vi "MGCC_MdlMgmt_MovetonewMicrogrid.vi"() -> ()   [LabVIEW 2016]
doc: "-----------------------------------------------------------------------------------------------------------------------\nCopyright <2019> <The University of Tennessee at Knoxville and the University of Tennessee Research Foundation>\nThis software is released under BSD-3 \nhttps://opensource.org/licenses/BSD-3-Clause \nAdditional license options available at https://utrf.tennessee.edu/industry/sample-agreements/\n-----------------------------------------------------------------------------------------------------------------------"
uses:
  Global_MdlMgmt.vi
  <vilib>/imath/engines/lvmath2/RunTimeEngine/IndexRead/NIMS M($,R2).vi
  <instcachedir>/0/NIMS M($,R2)_D9380E19261A4ADFB2D364AF6959C6EF.lvgen/NIMS M($,R2)_D9380E19261A4ADFB2D364AF6959C6EF_001.vi
  <vilib>/imath/engines/lvmath2/RunTimeEngine/BuiltInFunctions/max/1 input/NIMS_max(RM).vi
  <instcachedir>/0/NIMS_max(RM)_358AE92FF7FA4D91BF0D9DEC69043403.lvgen/NIMS_max(RM)_358AE92FF7FA4D91BF0D9DEC69043403_000.vi
  <vilib>/imath/engines/lvmath2/RunTimeEngine/BuiltInFunctions/max/1 input/NIMS_max(RV).vi
  <instcachedir>/0/NIMS_max(RV)_237633DB1D604D5BA7001287DF3C7957.lvgen/NIMS_max(RV)_237633DB1D604D5BA7001287DF3C7957_000.vi
  <vilib>/imathl/engines/lvmath/Functions/Error Handling/Create Error.vi
  <vilib>/imath/engines/lvmath2/RunTimeEngine/IndexRead/NIMS M($,S).vi
  <instcachedir>/0/NIMS M($,S)_3E5749BBB62E49528D4765A77F1F6D98.lvgen/NIMS M($,S)_3E5749BBB62E49528D4765A77F1F6D98_000.vi
  <vilib>/imath/engines/lvmath2/RunTimeEngine/BuiltInFunctions/length/NIMS_length(GV).vi
  <instcachedir>/0/NIMS_length(GV)_08A3D13377FD4E4B96F5795FBF3698FA.lvgen/NIMS_length(GV)_08A3D13377FD4E4B96F5795FBF3698FA_000.vi
  <instcachedir>/0/NIMS_length(GV)_08A3D13377FD4E4B96F5795FBF3698FA.lvgen/NIMS_length(GV)_08A3D13377FD4E4B96F5795FBF3698FA_002.vi
  <vilib>/imath/engines/lvmath2/RunTimeEngine/BuiltInFunctions/zeros/NIMS_M=zeros(I32,I32).vi
  <vilib>/imath/engines/lvmath2/RunTimeEngine/ErrorHandling/NIMS_Create Error From Enums.vi
  <vilib>/imath/engines/lvmath2/RunTimeEngine/IndexReplace/NIMS M(S,$)=V.vi
  <instcachedir>/0/NIMS M(S,$)=V_BCCFA522A894489B8FA760383D74A164.lvgen/NIMS M(S,$)=V_BCCFA522A894489B8FA760383D74A164_002.vi
  <vilib>/imath/engines/lvmath2/RunTimeEngine/BuiltInFunctions/zeros/NIMS_V=zeros(I32,I32).vi
  <vilib>/imath/engines/lvmath2/RunTimeEngine/RangeToken/NIMS_Range_R3 - Integer.vi
  <instcachedir>/0/NIMS_Range_R3 - Integer_A435E2FF893B4C718FD5055FE39FE2F6.lvgen/NIMS_Range_R3 - Integer_A435E2FF893B4C718FD5055FE39FE2F6_000.vi
  <vilib>/imath/engines/lvmath2/RunTimeEngine/CommandStatement/MC_CommandStatement_break.vi
  <vilib>/imath/engines/lvmath2/RunTimeEngine/IndexRead/NIMS M(S,R2).vi
  <instcachedir>/0/NIMS M(S,R2)_45730E4D0DB74D118F715F4F99DCE4D7.lvgen/NIMS M(S,R2)_45730E4D0DB74D118F715F4F99DCE4D7_000.vi
  <vilib>/imath/engines/lvmath2/RunTimeEngine/BuiltInFunctions/is_membermx/NIMS_is_membermx(GM,GM).vi
  <instcachedir>/0/NIMS_is_membermx(GM,GM)_DE25F6F493CE4EA1946032CBAF7A49B3.lvgen/NIMS_is_membermx(GM,GM)_DE25F6F493CE4EA1946032CBAF7A49B3_000.vi
  <vilib>/imath/engines/lvmath2/RunTimeEngine/BuiltInFunctions/sum/NIMS_sum(GM,Sca).vi
  <instcachedir>/0/NIMS_sum(GM,Sca)_79BF37D5D11844228B167097B6AFCFEB.lvgen/NIMS_sum(GM,Sca)_79BF37D5D11844228B167097B6AFCFEB_001.vi
  <vilib>/imath/engines/lvmath2/RunTimeEngine/IndexRead/NIMS M(S,S).vi
  <instcachedir>/0/NIMS M(S,S)_AC51E74150A542F7991B9634C66F3096.lvgen/NIMS M(S,S)_AC51E74150A542F7991B9634C66F3096_000.vi
  <vilib>/imath/engines/lvmath2/RunTimeEngine/IndexReplace/NIMS M(S,S)=S.vi
  <instcachedir>/0/NIMS M(S,S)=S_98E40400474E4398B113AE20298B4F82.lvgen/NIMS M(S,S)=S_98E40400474E4398B113AE20298B4F82_000.vi
  <vilib>/imath/engines/lvmath2/RunTimeEngine/BuiltInFunctions/sum/NIMS_sum(GV).vi
  <instcachedir>/0/NIMS_sum(GV)_67F5EC36BC034E54A6BEC5B0673C00E5.lvgen/NIMS_sum(GV)_67F5EC36BC034E54A6BEC5B0673C00E5_000.vi
  <vilib>/imath/engines/lvmath2/RunTimeEngine/BuiltInFunctions/findnz/NIMS_[1o]_findnz(GRowV).vi
  <instcachedir>/0/NIMS_[1o]_findnz(GRowV)_1AF74843B4874134ADE908C0A4A72F3C.lvgen/NIMS_[1o]_findnz(GRowV)_1AF74843B4874134ADE908C0A4A72F3C_000.vi
  <vilib>/imath/engines/lvmath2/RunTimeEngine/IndexRead/NIMS M($,V).vi
  <instcachedir>/0/NIMS M($,V)_706F2CE2C8E141269FD4C8A402E169C5.lvgen/NIMS M($,V)_706F2CE2C8E141269FD4C8A402E169C5_005.vi
  <vilib>/imath/engines/lvmath2/RunTimeSupport/NIMS_Get Any Vector_w Error - Matrix.vi
  <instcachedir>/0/NIMS_Get Any Vector_w Error - Matrix_2B7BCBEFD1FA4E1C95EFF9244314B21B.lvgen/NIMS_Get Any Vector_w Error - Matrix_2B7BCBEFD1FA4E1C95EFF9244314B21B_001.vi
  <vilib>/imath/engines/lvmath2/RunTimeEngine/BuiltInFunctions/sets_union/NIMS_sets_union(GV2).vi
  <instcachedir>/0/NIMS_sets_union(GV2)_D04DE11E528744D2B40881BC08732835.lvgen/NIMS_sets_union(GV2)_D04DE11E528744D2B40881BC08732835_007.vi
  <vilib>/imath/engines/lvmath2/RunTimeEngine/IndexReplace/NIMS M($,V)=V.vi
  <instcachedir>/0/NIMS M($,V)=V_456DED019FC24BEA8A1C4EECB3220DB5.lvgen/NIMS M($,V)=V_456DED019FC24BEA8A1C4EECB3220DB5_000.vi
  <vilib>/imath/engines/lvmath2/RunTimeEngine/RangeToken/NIMS_Range.vi
  <instcachedir>/0/NIMS_Range_A7C094595B484CA7AF10685B02D808ED.lvgen/NIMS_Range_A7C094595B484CA7AF10685B02D808ED_001.vi
  <vilib>/imath/engines/lvmath2/RunTimeEngine/NodeEndStatement/NIMS_NodeEndStatement_Output.vi
  <instcachedir>/0/NIMS_NodeEndStatement_Output_53EC0D466D134D7ABD903AC30B43404B.lvgen/NIMS_NodeEndStatement_Output_53EC0D466D134D7ABD903AC30B43404B_002.vi
  <instcachedir>/0/NIMS_NodeEndStatement_Output_53EC0D466D134D7ABD903AC30B43404B.lvgen/NIMS_NodeEndStatement_Output_53EC0D466D134D7ABD903AC30B43404B_011.vi
  <vilib>/imath/engines/lvmath2/RunTimeEngine/ErrorHandling/NIMS_Finalize Error.vi
  <vilib>/Utility/error.llb/Error Cluster From Error Code.vi
  <vilib>/ErrorRing/Error Ring.xnode
panel:
  out "Nodematrix":dbl[][](array[numeric])
  out "island_number":i32
  out "Microgrid Topology Overall":dbl[][](array[numeric])
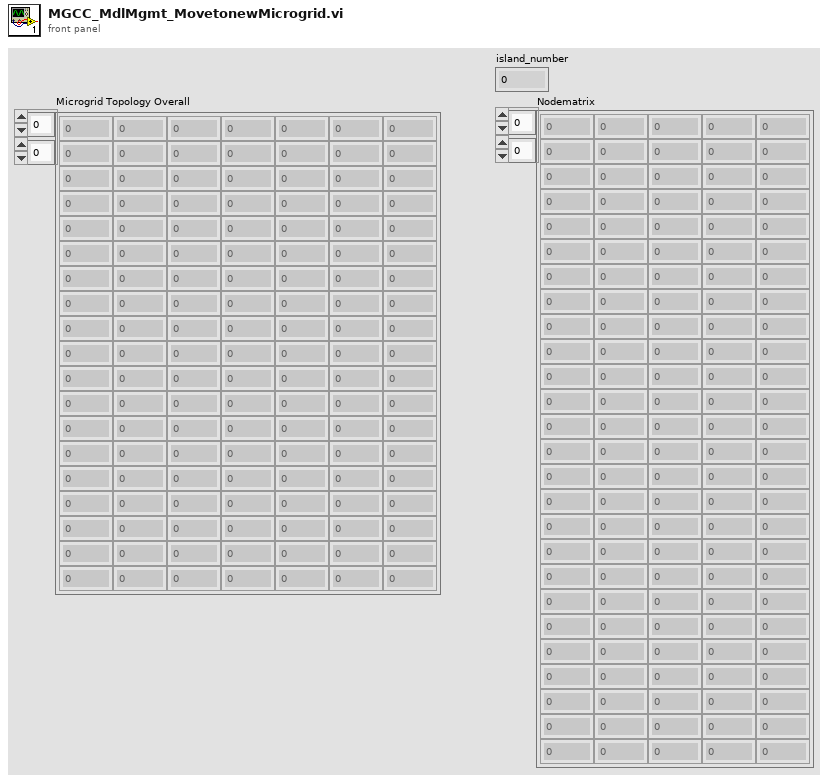
[diagram p1: front panel]
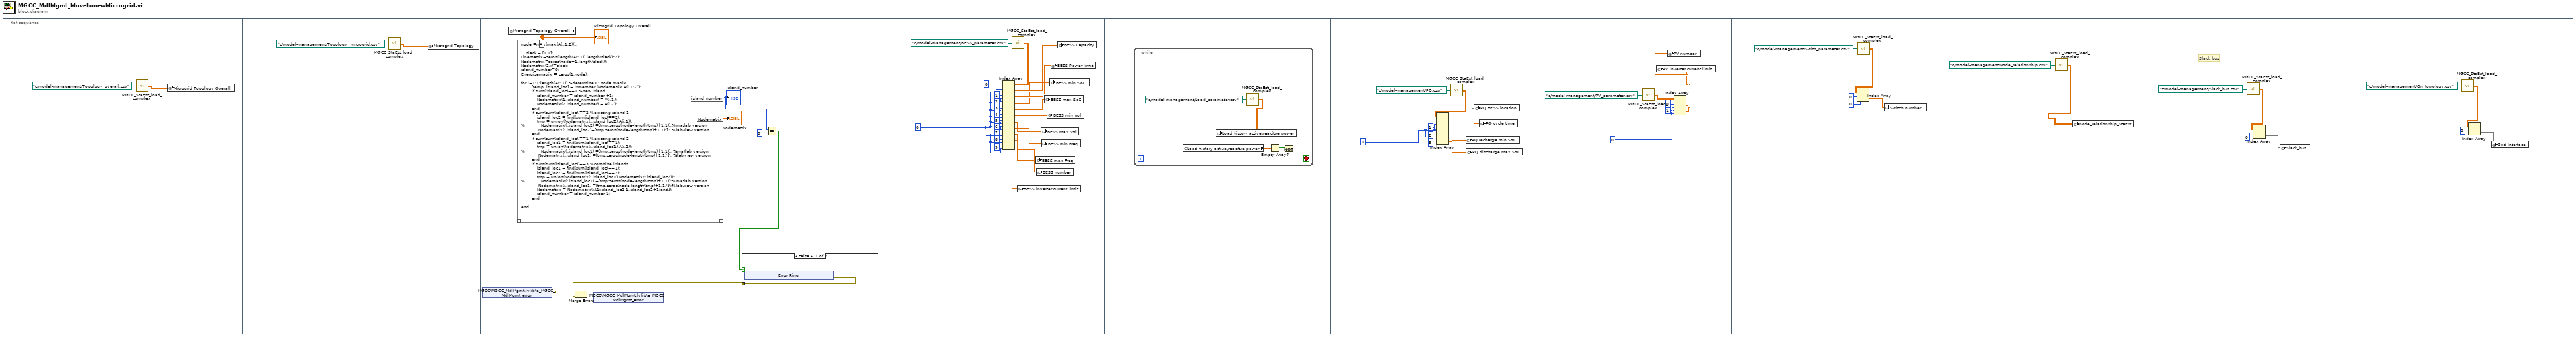
[diagram p0: block diagram]
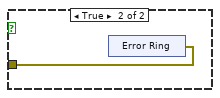
[diagram p2: hidden frame]
diagram:
  n1 = flat-sequence {
    frame #0 {
      n2 = call "MGCC_StaEst_load_complex.vi"("file path (dialog if empty)"=path "c:/model-management/Topology_overall.csv" ("file path (use dialog)")) -> ("Array 13"=w1:cdb[][])
      n3 = global write "Global_MdlMgmt.vi" "Microgrid Topology Overall"(w1) -> ()
    }
    frame #1 {
      n4 = call "MGCC_StaEst_load_complex.vi"("file path (dialog if empty)"=path "c:/model-management/Topology _microgrid.csv" ("file path (use dialog)")) -> ("Array 13"=w3:cdb[][])
      n5 = global write "Global_MdlMgmt.vi" "Microgrid Topology"(w3) -> ()
    }
    frame #2 {
      n6 = shared-variable "MGCC\\MGCC_MdlMgmt.lvlib\\e_MGCC_MdlMgmt_error"() -> (w10:errorcluster)  [unwired: 1 in, 1 out]
      n7 = global read "Global_MdlMgmt.vi" "Microgrid Topology Overall"() -> (w12:dbl[][])
      "Microgrid Topology Overall" <- w12
      n8 = mathscript code="node =max(max(A(:,1:2)));\n\n    slack = [0 0];\nLinematrix=zeros(length(A(:,1)),length(slack)*2);\nNodematrix=zeros(node+1,length(slack));\nNodematrix(2,:)=slack;\nisland_number=0;\nEnergizematrix = zeros(1,node);\n\nfor i=1:1:length(A(:,1)) %determine C: node matrix\n        [temp, island_loc] = ismember (Nodematrix,A(i,1:2));\n        if sum(island_loc)==0 %new island\n            island_number = island_number +1;\n            Nodematrix(1,island_number) = A(i,1);\n            Nodematrix(2,island_number) = A(i,2);\n        end\n        if sum(sum(island_loc))==2 %existing island 1\n            island_loc2 = find(sum(island_loc)==2);\n            tmp = union(Nodematrix(:,island_loc2),A(i,1));\n%            Nodematrix(:,island_loc2) =[tmp;zeros(node-length(tmp)+1,1)];%matlab version\n             Nodematrix(:,island_loc2)=[tmp,zeros(node-length(tmp)+1,1)']'; %labview version\n        end\n        if sum(sum(island_loc))==1 %existing island 2\n            island_loc1 = find(sum(island_loc)==1);\n            tmp = union(Nodematrix(:,island_loc1),A(i,2));\n%            Nodematrix(:,island_loc1) =[tmp;zeros(node-length(tmp)+1,1)]; %matlab version\n             Nodematrix(:,island_loc1) =[tmp,zeros(node-length(tmp)+1,1)']'; %labview version\n        end\n        if sum(sum(island_loc))==3 %combine islands\n            island_loc1 = find(sum(island_loc)==1);\n            island_loc2 = find(sum(island_loc)==2);\n            tmp = union(Nodematrix(:,island_loc1),Nodematrix(:,island_loc2));\n%            Nodematrix(:,island_loc1) =[tmp;zeros(node-length(tmp)+1,1)];%matlab version\n             Nodematrix(:,island_loc1) =[tmp,zeros(node-length(tmp)+1,1)']';%labview version\n            Nodematrix = Nodematrix(:,[1:island_loc2-1,island_loc2+1:end]);\n            island_number = island_number-1;\n        end\n\nend"("A"=w12) -> ("island_number"=w7:i32, "Nodematrix"=→"Nodematrix":dbl[][])  [unwired: 1 in, 1 out]
      "island_number" <- w7
      n9 = Equal?(x=w7, y=0) -> (x = y?=w5:bool)
      n10 = case shown="False" w5 {
        tunnel: [w13 w19] -> w8
        frame False {
          n11 = xnode "Error Ring"() -> ("error out"=w13:errorcluster)
        }
        frame True {
          n12 = xnode "Error Ring"() -> ("error out"=w19:errorcluster)
        }
      }
      n13 = Merge Errors(w10, w8) -> (w9:errorcluster)
      n14 = shared-variable "MGCC\\MGCC_MdlMgmt.lvlib\\e_MGCC_MdlMgmt_error"(w9) -> ()  [unwired: 1 in, 1 out]
    }
    frame #3 {
      w754 = 0
      n15 = call "MGCC_StaEst_load_complex.vi"("file path (dialog if empty)"=path "c:/model-management/BESS_parameter.csv" ("file path (use dialog)")) -> ("Array 13"=w764:cdb[][])
      n16 = Index Array(array=w764, index (row) #1=0 ("disabled index (row)"), index (col) #1=w754, index (row) #2=1 ("disabled index (row)"), index (col) #2=w754, index (row) #3=2 ("disabled index (row)"), index (col) #3=w754, index (row) #4=3 ("disabled index (row)"), index (col) #4=w754, index (row) #5=4 ("disabled index (row)"), index (col) #5=w754, index (row) #6=5 ("disabled index (row)"), index (col) #6=w754, index (row) #7=6 ("disabled index (row)"), index (col) #7=w754, index (row) #8=7 ("index (row)"), index (col) #8=w754, index (row) #9=8 ("index (row)"), index (col) #9=w754, index (row) #10=9 ("index (row)"), index (col) #10=w754) -> (element #1=w753:cdb, element #2=w752:cdb, element #3=w751:cdb, element #4=w750:cdb, element #5=w749:cdb, element #6=w748:cdb, element #7=w747:cdb, element #8=w746:cdb, element #9=w745:cdb, element #10=w744:cdb)
      n17 = global write "Global_MdlMgmt.vi" "BESS inverter current limit"(w744) -> ()
      n18 = global write "Global_MdlMgmt.vi" "BESS max Freq"(w746) -> ()
      n19 = global write "Global_MdlMgmt.vi" "BESS number"(w745) -> ()
      n20 = global write "Global_MdlMgmt.vi" "BESS max Vol"(w748) -> ()
      n21 = global write "Global_MdlMgmt.vi" "BESS min Freq"(w747) -> ()
      n22 = global write "Global_MdlMgmt.vi" "BESS max SoC"(w750) -> ()
      n23 = global write "Global_MdlMgmt.vi" "BESS min Vol"(w749) -> ()
      n24 = global write "Global_MdlMgmt.vi" "BESS min SoC"(w751) -> ()
      n25 = global write "Global_MdlMgmt.vi" "BESS Power limit"(w752) -> ()
      n26 = global write "Global_MdlMgmt.vi" "BESS Capacity"(w753) -> ()
    }
    frame #4 {
      n27 = while {
        stop <- w767 stop-if-true
        n28 = global read "Global_MdlMgmt.vi" "Load history active/reacitve power"() -> (w769:dbl[][])
        n29 = call "MGCC_StaEst_load_complex.vi"("file path (dialog if empty)"=path "c:/model-management/Load_parameter.csv" ("file path (use dialog)")) -> ("Array 13"=w770:cdb[][])
        n30 = global write "Global_MdlMgmt.vi" "Load history active/reacitve power"(w770) -> ()
        n31 = Empty Array?(array=w769) -> (empty?=w768:bool)
        n32 = Not(x=w768) -> (.not. x?=w767:bool)
      }
    }
    frame #5 {
      w780 = 0
      n33 = call "MGCC_StaEst_load_complex.vi"("file path (dialog if empty)"=path "c:/model-management/PQ.csv" ("file path (use dialog)")) -> ("Array 13"=w779:cdb[][])
      n34 = Index Array(array=w779, index (col) #1=w780, index (row) #2=1 ("disabled index (row)"), index (col) #2=w780, index (row) #3=2 ("disabled index (row)"), index (col) #3=w780, index (row) #4=3 ("disabled index (row)"), index (col) #4=w780) -> (element #1=w775:cdb[], element #2=w774:cdb, element #3=w773:cdb, element #4=w772:cdb)  [unwired: 1 in]
      n35 = global write "Global_MdlMgmt.vi" "PQ recharge min SoC"(w773) -> ()
      n36 = global write "Global_MdlMgmt.vi" "PQ discharge max SoC"(w772) -> ()
      n37 = global write "Global_MdlMgmt.vi" "PQ BESS location"(w775) -> ()
      n38 = global write "Global_MdlMgmt.vi" "PQ cycle time"(w774) -> ()
    }
    frame #6 {
      w786 = 0
      n39 = call "MGCC_StaEst_load_complex.vi"("file path (dialog if empty)"=path "c:/model-management/PV_parameter.csv" ("file path (use dialog)")) -> ("Array 13"=w787:cdb[][])
      n40 = Index Array(array=w787, index (row) #1=0 ("disabled index (row)"), index (col) #1=w786, index (row) #2=1 ("disabled index (row)"), index (col) #2=w786) -> (element #1=w783:cdb, element #2=w782:cdb)
      n41 = global write "Global_MdlMgmt.vi" "PV inverter current limit"(w782) -> ()
      n42 = global write "Global_MdlMgmt.vi" "PV number"(w783) -> ()
    }
    frame #7 {
      n43 = call "MGCC_StaEst_load_complex.vi"("file path (dialog if empty)"=path "c:/model-management/Swith_parameter.csv" ("file path (use dialog)")) -> ("Array 13"=w792:cdb[][])
      n44 = Index Array(array=w792, index (row)=0, index (col)=0 ("disabled index (col)")) -> (element=w789:cdb)
      n45 = global write "Global_MdlMgmt.vi" "Switch number"(w789) -> ()
    }
    frame #8 {
      n46 = call "MGCC_StaEst_load_complex.vi"("file path (dialog if empty)"=path "c:/model-management/Node_relationship.csv" ("file path (use dialog)")) -> ("Array 13"=w794:cdb[][])
      n47 = global write "Global_MdlMgmt.vi" "node_relationship_StaEst"(w794) -> ()
    }
    frame #9 {
      # "Slack_bus"
      n48 = call "MGCC_StaEst_load_complex.vi"("file path (dialog if empty)"=path "c:/model-management/Slack_bus.csv" ("file path (use dialog)")) -> ("Array 13"=w798:cdb[][])
      n49 = Index Array(array=w798, index (col)=0 ("disabled index (col)")) -> (element=w796:cdb[])  [unwired: 1 in]
      n50 = global write "Global_MdlMgmt.vi" "Slack_bus"(w796) -> ()
    }
    frame #10 {
      n51 = call "MGCC_StaEst_load_complex.vi"("file path (dialog if empty)"=path "c:/model-management/On_topology.csv" ("file path (use dialog)")) -> ("Array 13"=w802:cdb[][])
      n52 = Index Array(array=w802, index (row)=0) -> (element=w801:cdb[])  [unwired: 1 in]
      n53 = global write "Global_MdlMgmt.vi" "Grid Interface"(w801) -> ()
    }
  }
